vi "Create Event.vi"(8 "error in (no error)":errorcluster, 11 "OnChange_Boolean in":refnum<class "OnChangeNotifier_String.lvclass">) -> (0 "error out":errorcluster, 3 "OnChange_Boolean out":refnum<class "OnChangeNotifier_String.lvclass">)   [LabVIEW 2021, in "OnChangeNotifier_String.lvclass"]
uses:
  OnChangeNotifier_String.lvclass
  Support/Type.ctl
  OnChangeNotifier_String.lvclass/OnChangeNotifier_String.ctl
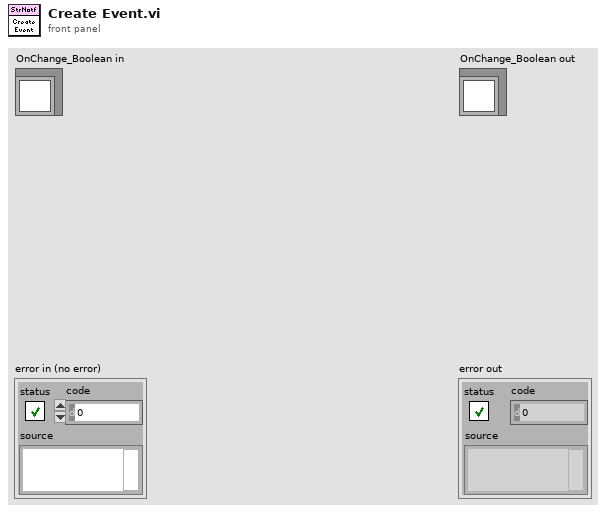
[diagram p1: front panel]
types:
  T1 = typedef "OnChangeNotifier_String.lvclass/Type.ctl" = string
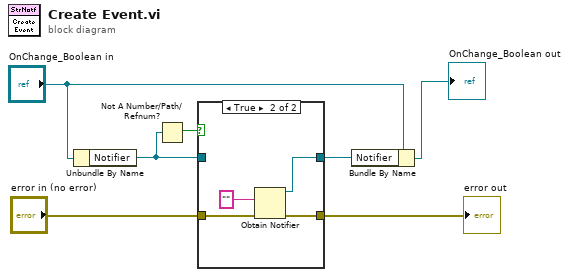
[diagram p0: block diagram]
diagram:
  n1 = Unbundle By Name("OnChange_Boolean in") -> ("Notifier"=w2:refnum<notifier>)
  n2 = Not A Number/Path/Refnum?(number/path/refnum=w2) -> (NaN/Path/Refnum?=w1:bool)
  n3 = case shown="True" w1 {
    tunnel: "error in (no error)" -> [w8 w13]
    tunnel: [w8 w12] -> w5
    tunnel: [w9 w11] -> w3
    tunnel: w2 -> [w9 _]
    frame False {
    }
    frame True {
      n4 = Obtain Notifier(notification data type=T1 "" ("Value"), error in (no error)=w13) -> (notifier out=w11:refnum<notifier>, error out=w12:errorcluster)  [unwired: 2 in, 1 out]
    }
  }
  "error out" <- w5
  n5 = Bundle By Name(cluster="OnChange_Boolean in", "Notifier"=w3) -> (→"OnChange_Boolean out":refnum<class "OnChangeNotifier_String.lvclass">)
